vi "Write Transfer Delivery Notifier.vi"(8 "error in (no error)":errorcluster, 10 "Transfer Delivery Notifier":refnum<notifier>, 11 "Turbo in":refnum<class "Turbo.lvclass">) -> (0 "error out":errorcluster, 3 "Turbo out":refnum<class "Turbo.lvclass">)   [LabVIEW 2015, in "cRIO-Carbondioxide.lvlib" / "CO2-Actor.lvlib" / "Turbo.lvclass"]
uses:
  Turbo.lvclass
  <vilib>/ActorFramework/Time-Delayed Send Message/Time-Delay Override Options.ctl
  Turbo.lvclass/Turbo.ctl
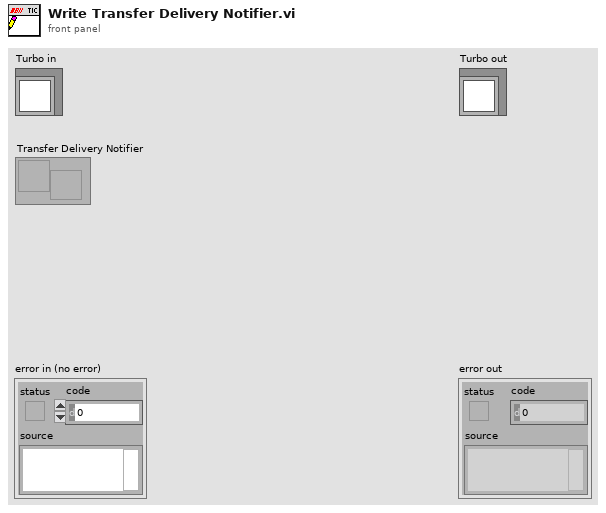
[diagram p1: front panel]
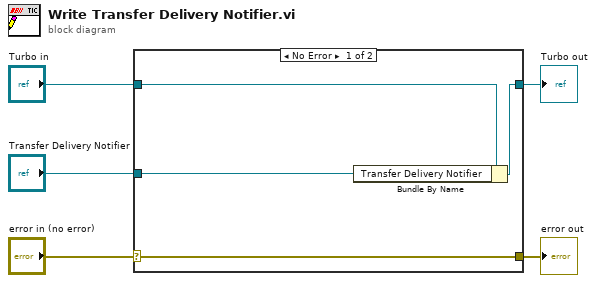
[diagram p0: block diagram]
diagram:
  n1 = case shown="No Error" "error in (no error)" {
    selector: "error in (no error)" -> [w9 w10]
    tunnel: [w9 w10] -> w4
    tunnel: [w7 w11] -> w2
    tunnel: "Turbo in" -> [w8 w11]
    tunnel: "Transfer Delivery Notifier" -> [w6 _]
    frame No Error {
      n2 = Bundle By Name(cluster=w8, "Transfer Delivery Notifier"=w6) -> (w7:refnum<class "Turbo.lvclass">)
    }
    frame Error {
    }
  }
  "error out" <- w4
  "Turbo out" <- w2
